vi "Configure Bus Source (AUDIO - Type).vi"(0 "VISA resource name":refnum<visa-resource-name>, 1 "Bit Order (0: LSB)":u16(ring) items=["LSB", "MSB"], 2 "Frame Size (8)":i32=8, 5 "BUS Number (9: Bus 1)":u16(ring)=9 items=["Bus 1"=9, "Bus 2"=10, "Bus 3"=11, "Bus 4"=12], 7 "Audio Bus Type (0: I2S)":u16(ring) items=["I2S", "Left Justified", "Right Justified", "Time-division multiplexing"], 9 "Delay Bits (1)":i32=1, 11 "error in (no error)":errorcluster, 12 "Channel Size (8)":i32=8) -> (4 "VISA resource name out":refnum<visa-resource-name>, 15 "error out":errorcluster)   [LabVIEW 2009, in "Tektronix DPO MSO 2000 4000 Series.lvlib"]
doc: "Conifgures Audio Bus type.\n\n<B>Note:</B> This VI is only valid if you have installed the AUDIO application module."
uses:
  <instrlib>/Tektronix DPO MSO 2000 4000 Series/Tektronix DPO MSO 2000 4000 Series.lvlib
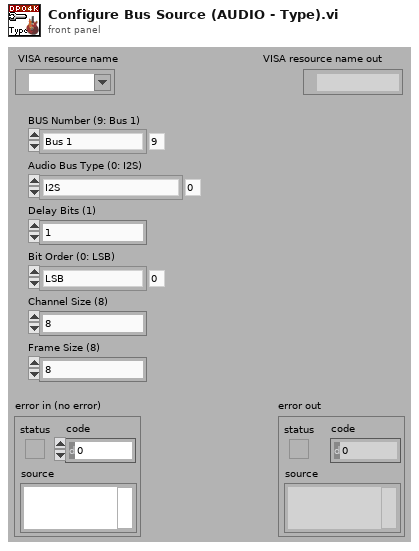
[diagram p1: front panel]
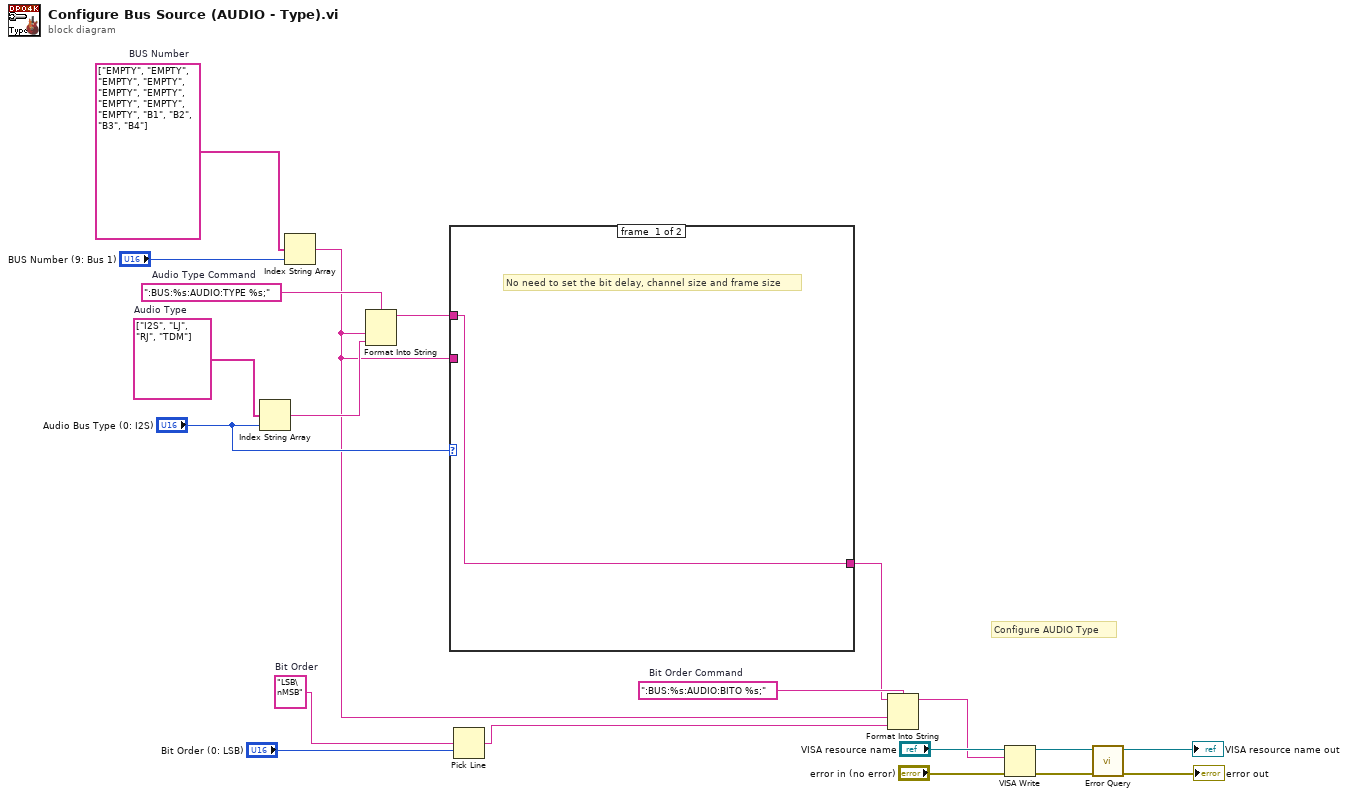
[diagram p0: block diagram]
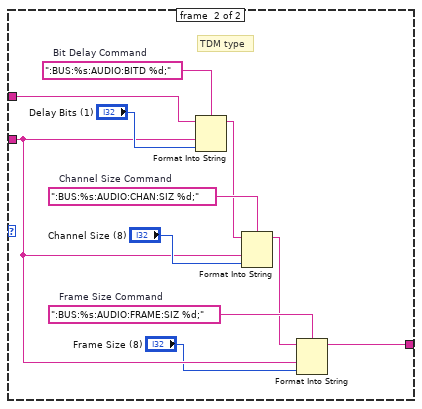
[diagram p2: hidden frame]
diagram:
  w13 = "LSB\nMSB"  # Bit Order
  w11 = ":BUS:%s:AUDIO:BITO %s;"  # Bit Order Command
  w17 = string[] ["I2S", "LJ", "RJ", "TDM"]  # Audio Type
  w18 = ":BUS:%s:AUDIO:TYPE %s;"  # Audio Type Command
  w19 = string[] ["EMPTY", "EMPTY", "EMPTY", "EMPTY", "EMPTY", "EMPTY", "EMPTY", "EMPTY", "EMPTY", "B1", "B2", "B3", "B4"]  # BUS Number
  # "Configure AUDIO Type"
  n1 = Index String Array(1:"Audio Bus Type (0: I2S)", 2:w17) -> (0:w16:string)  [unwired: 1 in]
  n2 = Index String Array(1:"BUS Number (9: Bus 1)", 2:w19) -> (0:w2:string)  [unwired: 1 in]
  n3 = Format Into String(format string=w18, w2, w16) -> (resulting string=w14:string)  [unwired: 2 in, 1 out]
  n4 = case shown="3, Default" "Audio Bus Type (0: I2S)" {
    tunnel: w2 -> [_ w26]
    tunnel: w14 -> [w21 w30]
    tunnel: [w21 w22] -> w10
    frame #0 {
      # "No need to set the bit delay, channel size and frame size"
    }
    frame #1 {
      w25 = ":BUS:%s:AUDIO:FRAME:SIZ %d;"  # Frame Size Command
      w29 = ":BUS:%s:AUDIO:CHAN:SIZ %d;"  # Channel Size Command
      w32 = ":BUS:%s:AUDIO:BITD %d;"  # Bit Delay Command
      # "TDM type"
      n5 = Format Into String(format string=w32, initial string=w30, w26, "Delay Bits (1)") -> (resulting string=w28:string)  [unwired: 1 in, 1 out]
      n6 = Format Into String(format string=w29, initial string=w28, w26, "Channel Size (8)") -> (resulting string=w23:string)  [unwired: 1 in, 1 out]
      n7 = Format Into String(format string=w25, initial string=w23, w26, "Frame Size (8)") -> (resulting string=w22:string)  [unwired: 1 in, 1 out]
    }
  }
  n8 = Pick Line(multi-line string=w13, line index="Bit Order (0: LSB)") -> (output string=w1:string)  [unwired: 1 in]
  n9 = Format Into String(format string=w11, initial string=w10, w2, w1) -> (resulting string=w7:string)  [unwired: 1 in, 1 out]
  n10 = VISA Write(VISA resource name="VISA resource name", write buffer=w7, error in (no error)="error in (no error)") -> (VISA resource name out=w6:refnum<visa-resource-name>, error out=w5:errorcluster)  [unwired: 1 out]
  n11 = call <instrlib>:"Error Query.vi"("error in (no error)"=w5, "VISA resource name"=w6) -> ("error out"=→"error out":errorcluster, "VISA resource name out"=→"VISA resource name out":refnum<visa-resource-name>)  [unwired: 6 in, 2 out]
